vi "StartGeneration1212(Host).vi"(1 "SYNC":bool, 2 "Channel Cluster":cluster{"CH1 ON ":bool, "CH2 ON":bool}, 3 "error in":errorcluster, 4 "resource name":T1="RIO0" caption="RIO Device") -> (0 "error out":errorcluster)   [LabVIEW 2018]
uses:
  <vilib>/userdefined/High Color/nirio_resource_hc.ctl
  <vilib>/Utility/error.llb/Error Cluster From Error Code.vi
  <vilib>/rvi/errors/niLvFpgaAdjustHostInterfaceError.vi
  <vilib>/FPGAPlugInAG/Dynamic/niLvFpga_Close_Dynamic.vi
  <vilib>/rvi/interface/nirviReadWriteControl/nirviReadWriteControl.xnode
  <vilib>/rvi/interface/nirviCloseFPGA/nirviCloseFPGA.xnode
  <vilib>/rvi/interface/Simulation/niFpgaSimulationCallBeginRW.vi
  NiFpgaLv.dll
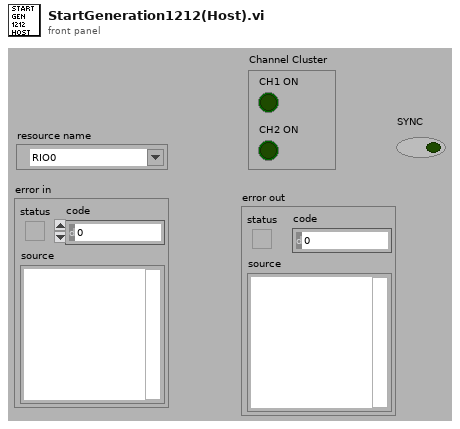
[diagram p1: front panel]
types:
  T1 = typedef "nirio_resource_hc.ctl" = tag
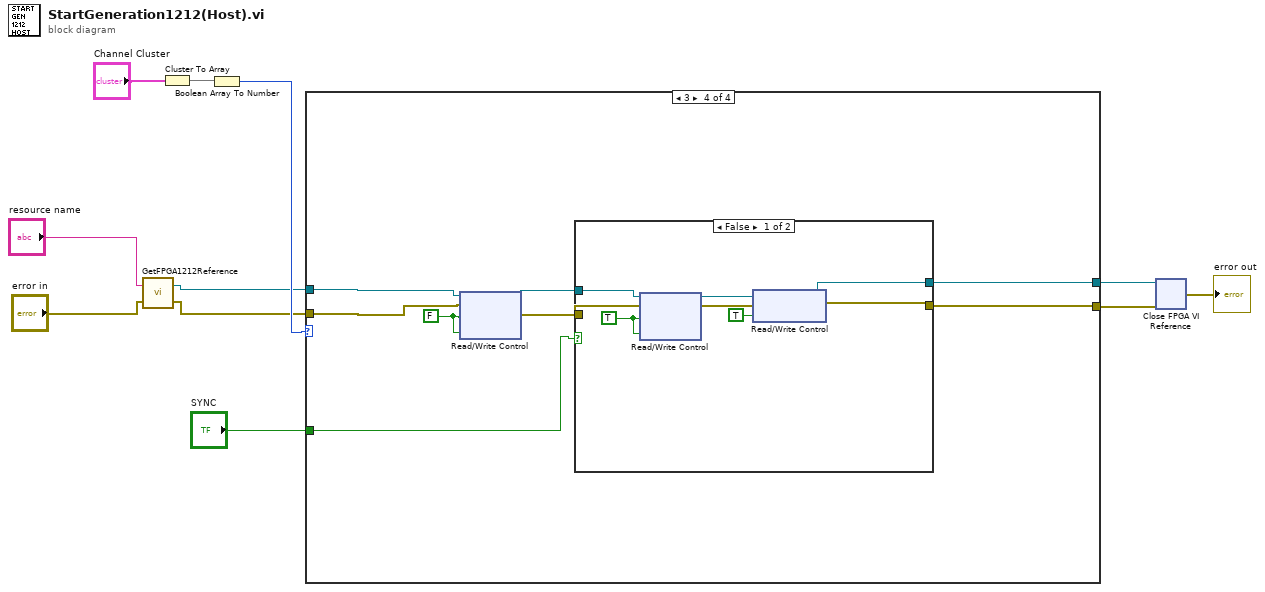
[diagram p0: block diagram]
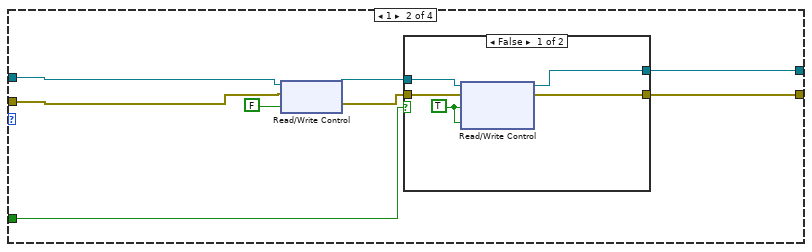
[diagram p3: hidden frame]
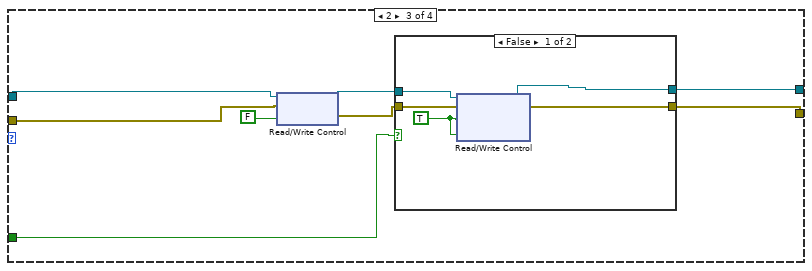
[diagram p5: hidden frame]
diagram:
  n1 = call "GetFPGA1212Reference.vi"("error in"="error in", "RIO Device IN"="resource name") -> ("error out"=w1:errorcluster, "FPGA VI Reference Out"=w2:refnum<k20>)
  n2 = Cluster To Array(cluster="Channel Cluster") -> (array=w8:bool[])
  n3 = Boolean Array To Number(Boolean array=w8) -> (number=w6:u32)
  n4 = case shown="3" w6 {
    tunnel: [w12 w16 w31 w46] -> w10
    tunnel: [w13 w19 w34 w49] -> w9
    tunnel: w2 -> [w13 w18 w33 w48]
    tunnel: w1 -> [w12 w17 w32 w47]
    tunnel: "SYNC" -> [_ w15 w30 w45]
    frame 0, Default {
    }
    frame 1 {
      n5 = xnode "Read/Write Control"("FPGA VI Reference In"=w18, "error in"=w17, "EN_CH0"=FALSE ("START")) -> ("FPGA VI Reference Out"=w21:refnum<k20>, "error out"=w20:errorcluster)
      n6 = case shown="False" w15 {
        tunnel: w21 -> [w26 w28]
        tunnel: w20 -> [w25 w27]
        tunnel: [w24 w28] -> w19
        tunnel: [w23 w27] -> w16
        frame False {
          w22 = TRUE ("START_CH1")
          n7 = xnode "Read/Write Control"("FPGA VI Reference In"=w26, "error in"=w25, "EN_CH0"=w22, "START_CH"=w22) -> ("FPGA VI Reference Out"=w24:refnum<k20>, "error out"=w23:errorcluster)
        }
        frame True {
        }
      }
    }
    frame 2 {
      n8 = xnode "Read/Write Control"("FPGA VI Reference In"=w33, "error in"=w32, "EN_CH1"=FALSE ("START")) -> ("FPGA VI Reference Out"=w36:refnum<k20>, "error out"=w35:errorcluster)
      n9 = case shown="False" w30 {
        tunnel: w36 -> [w41 w43]
        tunnel: w35 -> [w40 w42]
        tunnel: [w39 w43] -> w34
        tunnel: [w38 w42] -> w31
        frame False {
          w37 = TRUE ("START_CH1")
          n10 = xnode "Read/Write Control"("FPGA VI Reference In"=w41, "error in"=w40, "EN_CH1"=w37, "START_CH"=w37) -> ("FPGA VI Reference Out"=w39:refnum<k20>, "error out"=w38:errorcluster)
        }
        frame True {
        }
      }
    }
    frame 3 {
      w44 = FALSE ("START")
      n11 = xnode "Read/Write Control"("FPGA VI Reference In"=w48, "error in"=w47, "EN_CH1"=w44, "EN_CH0"=w44) -> ("FPGA VI Reference Out"=w51:refnum<k20>, "error out"=w50:errorcluster)
      n12 = case shown="False" w45 {
        tunnel: w51 -> [w59 w61]
        tunnel: w50 -> [w58 w60]
        tunnel: [w55 w61] -> w49
        tunnel: [w54 w60] -> w46
        frame False {
          w53 = TRUE ("START_CH1")
          n13 = xnode "Read/Write Control"("FPGA VI Reference In"=w59, "error in"=w58, "EN_CH1"=w53, "EN_CH0"=w53) -> ("FPGA VI Reference Out"=w57:refnum<k20>, "error out"=w56:errorcluster)
          n14 = xnode "Read/Write Control"("FPGA VI Reference In"=w57, "error in"=w56, "START_CH"=TRUE) -> ("FPGA VI Reference Out"=w55:refnum<k20>, "error out"=w54:errorcluster)
        }
        frame True {
        }
      }
    }
  }
  n15 = xnode "Close FPGA VI Reference"("FPGA VI Reference In"=w9, "error in"=w10) -> ("error out"=→"error out":errorcluster)
